vi "Sample_SimpleNumericRead.vi"() -> ()   [LabVIEW 2022 SP3]
panel:
  out "data":i32
  out "RData":variant
  out "Read status?":bool
  in  "String":string
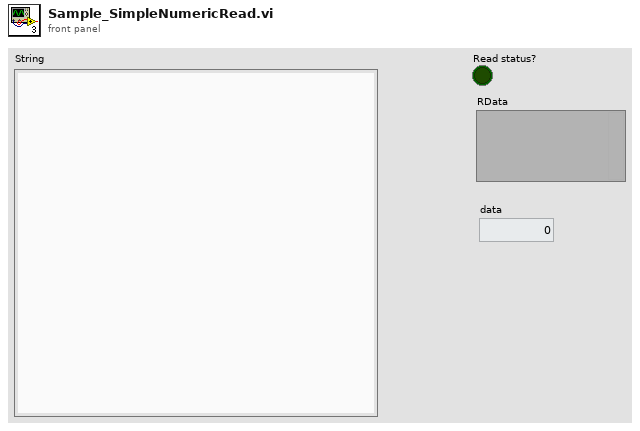
[diagram p1: front panel]
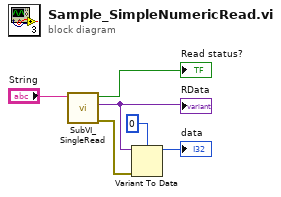
[diagram p0: block diagram]
diagram:
  n1 = call "SubVI_SingleRead.vi"("String"="String") -> ("error out"=w2:errorcluster, "RData"=w4:variant, "Read status?"=→"Read status?":bool)  [unwired: 7 in]
  "RData" <- w4
  n2 = Variant To Data(error in=w2, type=0, Variant=w4) -> (data=→"data":i32)  [unwired: 1 out]
